vi "DP-Calibrate.vi"(0 "state":T1, 1 "freq":dbl[](array[numeric]), 5 "flip":bool, 7 "Nominal Max SPLs":dbl[](array[numeric]), 9 "Acoustic System":string, 11 "error in (no error)":errorcluster, 12 "Override recal check?":bool) -> (4 "Max SPL1":dbl, 6 "Max SPL2":dbl, 15 "error out":errorcluster)   [LabVIEW 2020]
uses:
  Typedefs/DP-Runtime State.ctl
  epl-vi-lib/PXI DAQ VIs/AIDI/Typedefs/AIDI-Action.ctl
  epl-vi-lib/Utility VIs/Math VIs/FFTtoR,Theta (1D).VI
panel:
  in  "Averages":i32=4
  out "Mag graph":dbl[](graph)
  out "Mic Signal":dbl[](graph)
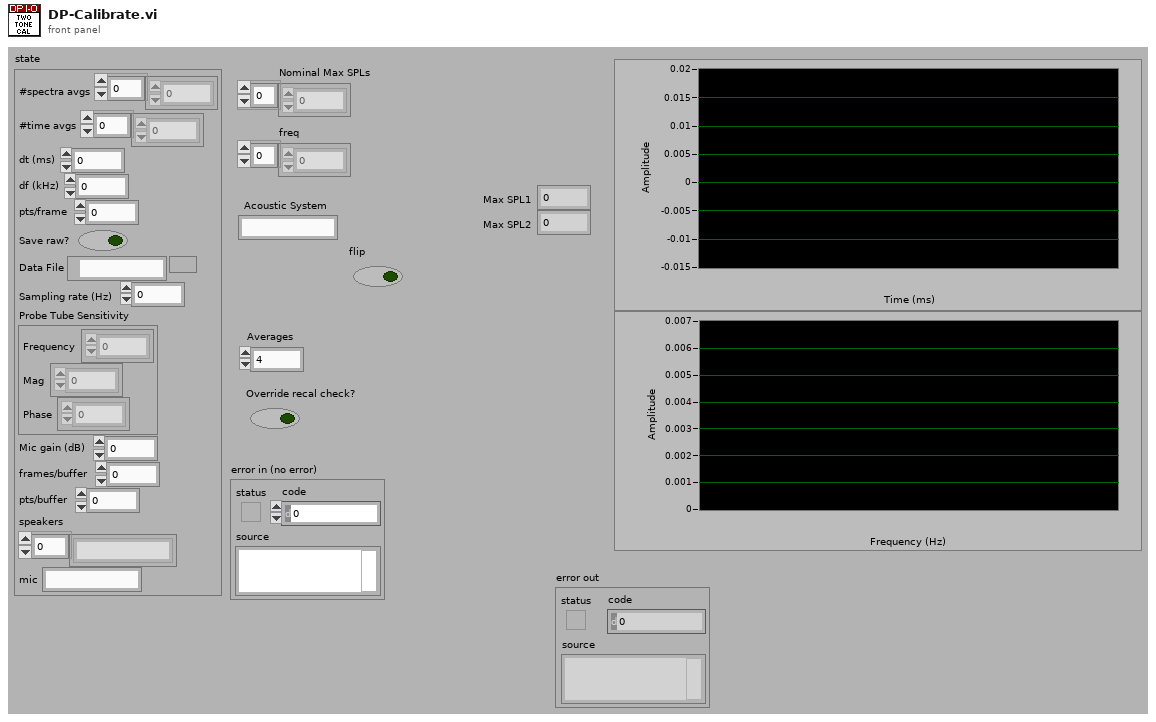
[diagram p1: front panel]
types:
  T1 = typedef "DP-Runtime State.ctl" = cluster{"#spectra avgs":i32[], "#time avgs":i32[], "dt (ms)":dbl, "df (kHz)":dbl, "pts/frame":i32, "Save raw?":bool, "Data File":path, "Sampling rate (Hz)":dbl, "Probe Tube Sensitivity":cluster{"Frequency":dbl[], "Mag":dbl[], "Phase":dbl[]}, "Mic gain (dB)":dbl, "frames/buffer":i32, "pts/buffer":i32, "speakers":string[], "mic":string}
  T2 = typedef "AIDI-Action.ctl" = enum16{"Configure", "Initialize", "Start", "Read", "Clean up", "Init & Start", "Config & Test", "Position", "Skip"}
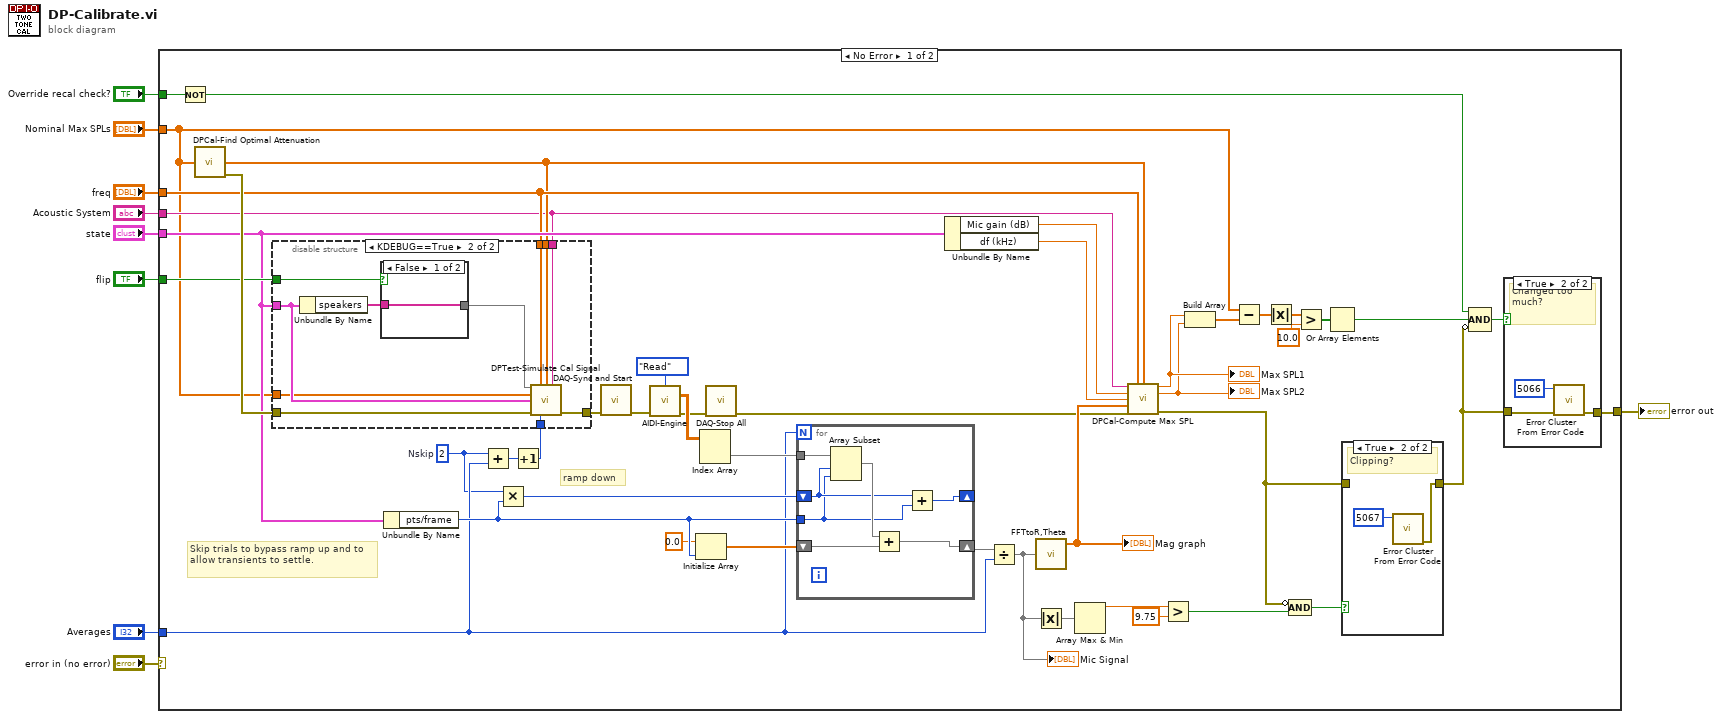
[diagram p0: block diagram]
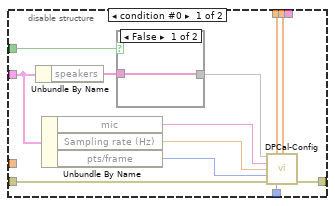
[diagram p2: hidden frame]
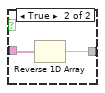
[diagram p3: hidden frame]
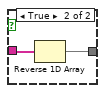
[diagram p4: hidden frame]
diagram:
  n1 = case shown="No Error" "error in (no error)" {
    selector: "error in (no error)" -> [_ w99]
    tunnel: [w44 w99] -> w8
    tunnel: "freq" -> [w17 _]
    tunnel: "Acoustic System" -> [w14 _]
    tunnel: "Nominal Max SPLs" -> [w13 _]
    tunnel: "Override recal check?" -> [w35 _]
    tunnel: "Averages" -> [w28 _]
    tunnel: "state" -> [w27 _]
    tunnel: "flip" -> [w33 _]
    frame No Error {
      w19 = 2  # Nskip
      # "ramp down"
      # "Skip trials to bypass ramp up and to allow transients to settle."
      n2 = Not(x=w35) -> (.not. x?=w34:bool)
      n3 = call "DPCal-Find Optimal Attenuation.vi"("Nominal Max SPL"=w13) -> ("Attenuation (dB)"=w16:dbl[], "error out"=w55:errorcluster)  [unwired: 13 in]
      n4 = Unbundle By Name(w27) -> ("pts/frame"=w29:i32)
      n5 = Add(x=w19, y=w28) -> (x+y=w22:i32)
      n6 = Multiply(x=w19, y=w29) -> (x*y=w30:i32)
      n7 = Increment(x=w22) -> (x+1=w20:i32)
      n8 = disable-structure shown="KDEBUG==True" {
        disable-tunnel: w55 -> [w67 w81]
        disable-tunnel: w33 -> [w66 w80]
        disable-tunnel: w27 -> [w65 w73]
        disable-tunnel: [w60 w77] -> w21
        disable-tunnel: w20 -> [w59 w76]
        disable-tunnel: w17 -> [w57 w75]
        disable-tunnel: w16 -> [w56 w74]
        disable-tunnel: w14 -> [_ w72]
        disable-tunnel: w13 -> [_ w71]
        frame condition #0 {
          n9 = Unbundle By Name(w65) -> ("speakers"=w64:string[])
          n10 = Unbundle By Name(w65) -> ("mic"=w62:string, "Sampling rate (Hz)"=w61:dbl, "pts/frame"=w58:i32)
          n11 = case shown="False" w66 {
            tunnel: w64 -> [w68 w70]
            tunnel: [w68 w69] -> w63
            frame False {
            }
            frame True {
              n12 = Reverse 1D Array(array=w70) -> (reversed array=w69:string[])
            }
          }
          n13 = call "DPCal-Config.vi"("Speakers"=w63, "freqs"=w57, "Attenuation (dB)"=w56, "Mic"=w62, "Sampling Rate (Hz)"=w61, "Npts"=w58, "error in (no error)"=w67, "Nbuf"=w59) -> ("error out"=w60:errorcluster)  [unwired: 7 in]
        }
        frame condition #1 (active) {
          n14 = Unbundle By Name(w73) -> ("speakers"=w79:string[])
          n15 = case shown="False" w80 {
            tunnel: w79 -> [w82 w84]
            tunnel: [w82 w83] -> w78
            frame False {
            }
            frame True {
              n16 = Reverse 1D Array(array=w84) -> (reversed array=w83:string[])
            }
          }
          n17 = call "DPTest-Simulate Cal Signal.vi"("Speakers"=w78, "freqs"=w75, "Attenuation (dB)"=w74, "Acoustic system"=w72, "ceilings"=w71, "state"=w73, "error in (no error)"=w81, "Nbuf"=w76) -> ("error out"=w77:errorcluster)  [unwired: 7 in]
        }
      }
      n18 = call "DAQ-Sync and Start.vi"("error in (no error)"=w21) -> ("error out"=w10:errorcluster)  [unwired: 14 in]
      n19 = call "AIDI-Engine.vi"("Action"=AIDI-Action."Read", "error in (no error)"=w10) -> ("AI"=w12:dbl[][], "error out"=w11:errorcluster)  [unwired: 8 in, 4 out]
      n20 = Initialize Array(0.0, w29) -> (w31:dbl[])
      n21 = Index Array(array=w12) -> (element=w32:dbl[])  [unwired: 2 in]
      n22 = call "DAQ-Stop All.vi"("error in (no error)"=w11) -> ("error out"=w23:errorcluster)  [unwired: 14 in]
      n23 = for {
        N: w28 -> [_]
        shift-right: [w88] -> w54
        shift-left: w31 -> [w90]
        tunnel: w32 -> [w91]
        shift-right: [w85] -> _
        shift-left: w30 -> [w87]
        tunnel: w29 -> [w86]
        n24 = Array Subset(array=w91, index=w87, length=w86) -> (w89:dbl[])
        n25 = Add(x=w89, y=w90) -> (x+y=w88:dbl[])
        n26 = Add(x=w87, y=w86) -> (x+y=w85:i32)
      }
      n27 = Unbundle By Name(w27) -> ("Mic gain (dB)"=w26:dbl, "df (kHz)"=w25:dbl)
      n28 = Divide(x=w54, y=w28) -> (x/y=w43:dbl[])
      "Mic Signal" <- w43
      n29 = call-poly "FFTtoR,Theta.VI"("X"=w43) -> ("+Freq. Mag of FFT"=w24:dbl[])  [unwired: 1 in, 1 out]
      "Mag graph" <- w24
      n30 = Absolute Value(x=w43) -> (abs(x)=w42:dbl[])
      n31 = Array Max & Min(array=w42) -> (max value=w41:dbl)  [unwired: 3 out]
      n32 = call "DPCal-Compute Max SPL.vi"("Acoustic System"=w14, "freqs"=w17, "Attenuation (dB)"=w16, "Probe mic gain (dB)"=w26, "df (kHz)"=w25, "Magnitude"=w24, "error in (no error)"=w23) -> ("Max SPL1"=w53:dbl, "Max SPL2"=w52:dbl, "error out"=w38:errorcluster)  [unwired: 6 in]
      "Max SPL1" <- w53
      "Max SPL2" <- w52
      n33 = Greater?(x=w41, y=9.75) -> (0:w39:bool)
      n34 = Build Array(w53, w52) -> (w51:dbl[])
      n35 = Subtract(x=w13, y=w51) -> (x-y=w50:dbl[])
      n36 = Absolute Value(x=w50) -> (abs(x)=w49:dbl[])
      n37 = Compound Arithmetic op=AND(invert w38, w39) -> (w36:bool)
      n38 = Greater?(x=w49, y=10.0) -> (0:w47:bool[])
      n39 = Or Array Elements(Boolean array=w47) -> (logical OR=w46:bool)
      n40 = case shown="True" w36 {
        tunnel: w38 -> [w92 _]
        tunnel: [w92 w93] -> w37
        frame False {
        }
        frame True {
          # "Clipping?"
          n41 = call <vilib>:"Error Cluster From Error Code.vi"("error code (0)"=5067) -> ("error out"=w93:errorcluster)  [unwired: 8 in]
        }
      }
      n42 = Compound Arithmetic op=AND(w34, w46, invert w37) -> (w45:bool)
      n43 = case shown="True" w45 {
        tunnel: w37 -> [w95 w98]
        tunnel: [w95 w96] -> w44
        frame False {
        }
        frame True {
          # "Changed too much?"
          n44 = call <vilib>:"Error Cluster From Error Code.vi"("error in (no error)"=w98, "error code (0)"=5066) -> ("error out"=w96:errorcluster)  [unwired: 7 in]
        }
      }
    }
    frame Error {
    }
  }
  "error out" <- w8
